vi "ProgMon.Set State.vi"(8 "error in":errorcluster, 10 "Remaining Secs":dbl=inf, 11 "Action":T1=enum."Set Rem Secs") -> (0 "error out":errorcluster)   [LabVIEW 2024, in "EQMF.lvlib" / "Status Utils.lvlib"]
uses:
  Status Utils.lvlib
  PrgMon.Action.ctl
  Queues/Queue Utils.lvlib
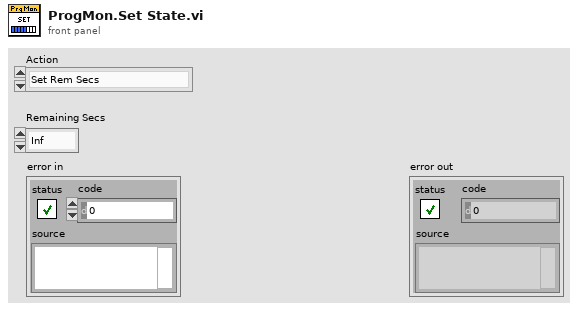
[diagram p1: front panel]
types:
  T1 = typedef "EQMF.lvlib/Status Utils.lvlib/PrgMon.Action.ctl" = enum16{"Reset", "Start", "Set Rem Secs", "Suspend", "Resume", "End"}
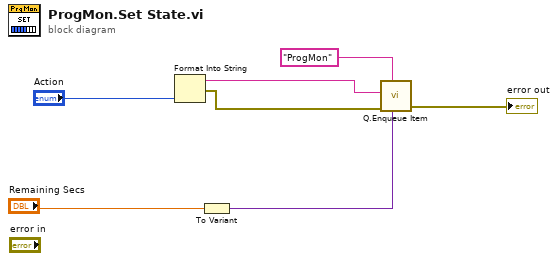
[diagram p0: block diagram]
diagram:
  n1 = Format Into String("Action") -> (resulting string=w4:string, error out=w3:errorcluster)  [unwired: 3 in]
  n2 = To Variant(anything="Remaining Secs") -> (Variant=w2:variant)
  n3 = call "Q.Enqueue Item.vi"("Data1"=w2, "Q Name"="ProgMon" ("name (unnamed)"), "Error In"=w3, "Cmd"=w4) -> ("error out"=→"error out":errorcluster)  [unwired: 6 in, 1 out]
